vi "Get value.vi"(0 "Stack in":refnum<class "Stack.lvclass">, 11 "error in (no error)":errorcluster) -> (3 "PUT Settings":T1, 4 "Stack out":refnum<class "Stack.lvclass">, 6 "Resolution Geometry":string, 10 "Assembly Settings":T1, 13 "Is real run":bool, 14 "Component Settings":T1, 15 "error out":errorcluster)   [LabVIEW 2021, in "Stack.lvclass"]
uses:
  Stack.lvclass
  Stack.lvclass/Stack.ctl
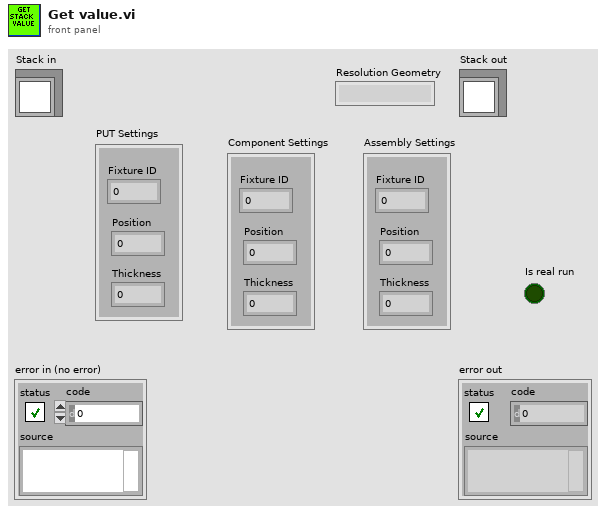
[diagram p1: front panel]
types:
  T1 = cluster{"Fixture ID":dbl, "Position":dbl, "Thickness":dbl}
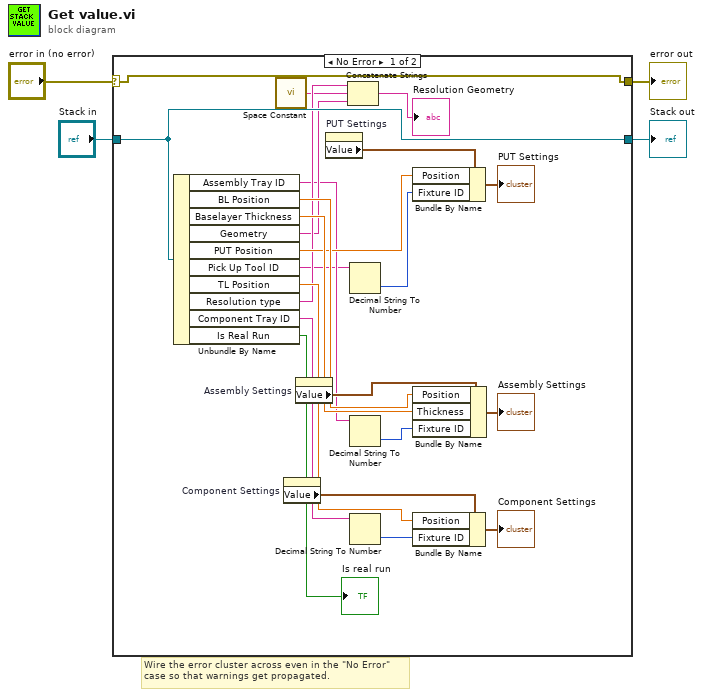
[diagram p0: block diagram]
diagram:
  # "Wire the error cluster across even in the \"No Error\"\ncase so that warnings get propagated."
  n1 = case shown="No Error" "error in (no error)" {
    selector: "error in (no error)" -> [w27 w29]
    tunnel: [w27 w29] -> w3
    tunnel: [w26 w28] -> w1
    tunnel: "Stack in" -> [w26 w28]
    frame No Error {
      n2 = Unbundle By Name(w26) -> ("Assembly Tray ID"=w11:string, "BL Position"=w22:dbl, "Baselayer Thickness"=w23:dbl, "Geometry"=w14:string, "PUT Position"=w17:dbl, "Pick Up Tool ID"=w7:string, "TL Position"=w16:dbl, "Resolution type"=w15:string, "Component Tray ID"=w10:string, "Is Real Run"=→"Is real run":bool)
      n3 = call <vilib>:"Space Constant.vi"() -> ("String"=w12:string)
      n4 = property on="Component Settings" class="Clust (strict)"() -> ("Value"=w21:T1)  [unwired: 2 in, 2 out]
      n5 = property on="Assembly Settings" class="Clust (strict)"() -> ("Value"=w24:T1)  [unwired: 2 in, 2 out]
      n6 = property on="PUT Settings" class="Clust (strict)"() -> ("Value"=w19:T1)  [unwired: 2 in, 2 out]
      n7 = Concatenate Strings(w15, w12, w14) -> (→"Resolution Geometry":string)
      n8 = Decimal String To Number(string=w7) -> (number=w8:i32)  [unwired: 2 in, 1 out]
      n9 = Decimal String To Number(string=w11) -> (number=w6:i32)  [unwired: 2 in, 1 out]
      n10 = Decimal String To Number(string=w10) -> (number=w9:i32)  [unwired: 2 in, 1 out]
      n11 = Bundle By Name(cluster=w19, "Position"=w17, "Fixture ID"=w8) -> (→"PUT Settings":T1)
      n12 = Bundle By Name(cluster=w24, "Position"=w22, "Thickness"=w23, "Fixture ID"=w6) -> (→"Assembly Settings":T1)
      n13 = Bundle By Name(cluster=w21, "Position"=w16, "Fixture ID"=w9) -> (→"Component Settings":T1)
    }
    frame Error {
    }
  }
  "error out" <- w3
  "Stack out" <- w1
